vi "Fake Data.vi"(11 "params":variant) -> (3 "data out":variant)   [LabVIEW 2020]
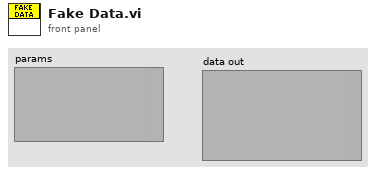
[diagram p1: front panel]
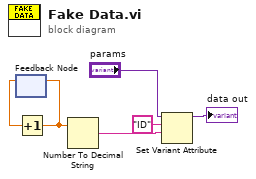
[diagram p0: block diagram]
diagram:
  n1 = feedback #1() -> (w6:dbl)  [unwired: 1 in]
  n2 = Increment(x=w6) -> (x+1=w5:dbl)
  n3 = feedback-in #1(w5) -> ()
  n4 = Number To Decimal String(number=w5) -> (decimal integer string=w3:string)  [unwired: 1 in]
  n5 = Set Variant Attribute(Variant="params", name="ID", value=w3) -> (Variant out=→"data out":variant)  [unwired: 1 in, 2 out]
